vi "initialize.vi"(8 "error in (no error)":errorcluster, 10 "action configuration":refnum<class "action configuration.lvclass">, 11 "Action in":refnum<class "action.lvclass">) -> (0 "error out":errorcluster, 2 "data allocations":T1, 3 "Action out":refnum<class "action.lvclass">)   [LabVIEW 2015, in "action.lvclass"]
doc: "Initializes the action based on the Action Configuration and returns a set of allocated channels."
uses:
  action.lvclass
  action configuration parent/action configuration.lvclass
  <vilib>/NI/Tag Bus Module Framework/channel/data tables.ctl
  <vilib>/NI/Tag Bus/dictionary/data dictionary.lvclass
  <vilib>/NI/Tag Bus/dictionary table pair.ctl
  <vilib>/NI/Tag Bus/table/data table.ctl
  <vilib>/NI/Tag Bus Module Framework/channel/TBM channel.lvclass
  <vilib>/NI/Tag Bus/table/data table.lvlib
  <vilib>/NI/Tag Bus/tag bus.lvlib
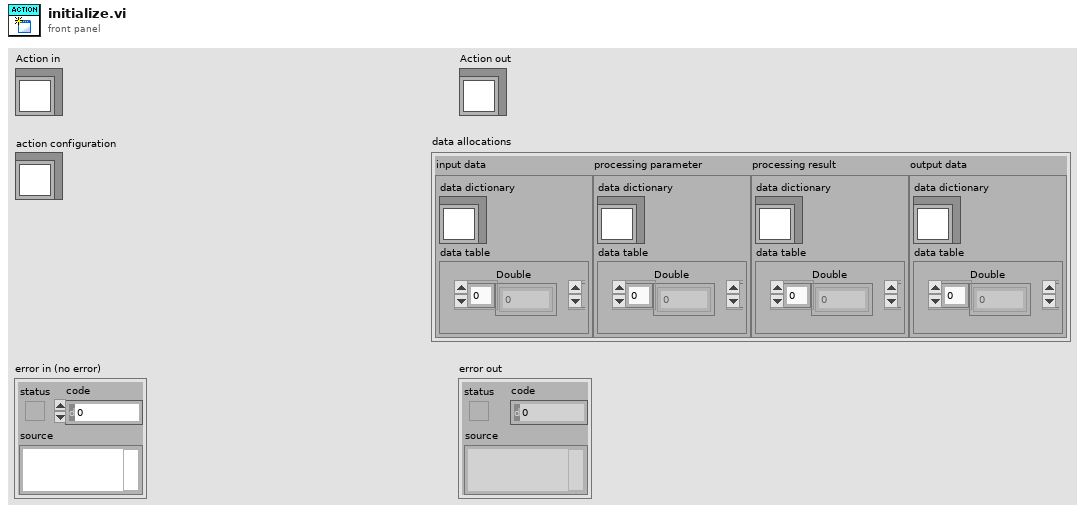
[diagram p1: front panel]
types:
  T1 = typedef "TBM channel.lvclass/data tables.ctl" = cluster{"input data":T2, "processing parameter":T2, "processing result":T2, "output data":T2}
  T2 = typedef "tag bus.lvlib/dictionary table pair.ctl" = cluster{"data dictionary":refnum<class "data dictionary.lvclass">, "data table":T3}
  T3 = typedef "tag bus.lvlib/data table.lvlib/data table.ctl" = cluster{"Double":dbl[], "Single":sgl[], "I64":i64[], "I32":i32[], "I16":i16[], "I8":i8[], "U64":u64[], "U32":u32[], "U16":u16[], "U8":u8[], "Boolean":bool[], "String":string[], "Array of Double":cluster{"DBL Array":dbl[]}[], "Array of Single":cluster{"SGL Array":sgl[]}[], "Array of I64":cluster{"I64 Array":i64[]}[], "Array of I32":cluster{"I32 Array":i32[]}[], "Array of I16":cluster{"I16 Array":i16[]}[], "Array of I8":cluster{"I8 Array":i8[]}[], "Array of U64":cluster{"U64 Array":u64[]}[], "Array of U32":cluster{"U32 Array":u32[]}[], "Array of U16":cluster{"U16 Array":u16[]}[], "Array of U8":cluster{"U8 Array":u8[]}[], "Array of Boolean":cluster{"Boolean Array":bool[]}[], "Array of String":cluster{"String Array":string[]}[]}
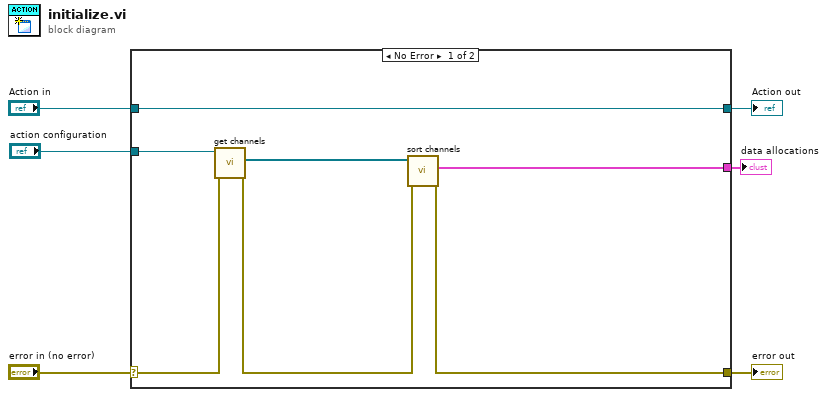
[diagram p0: block diagram]
diagram:
  n1 = case shown="No Error" "error in (no error)" {
    selector: "error in (no error)" -> [w10 w15]
    tunnel: [w8 w15] -> w5
    tunnel: [w13 w14] -> w3
    tunnel: "Action in" -> [w13 w14]
    tunnel: "action configuration" -> [w12 _]
    tunnel: [w7 _] -> w1
    frame No Error {
      n2 = call-dynamic "get channels.vi"("error in (no error)"=w10, "action configuration in"=w12) -> ("error out"=w9:errorcluster, "action channels"=w11:refnum<class "TBM channel.lvclass">[])  [unwired: 7 in, 1 out]
      n3 = call <vilib>:"sort channels.vi"("error in"=w9, "channels in"=w11) -> ("error out"=w8:errorcluster, "data allocations"=w7:T1)  [unwired: 7 in, 1 out]
    }
    frame Error {
    }
  }
  "error out" <- w5
  "Action out" <- w3
  "data allocations" <- w1
